vi "JSON Editor.vi"() -> ()   [LabVIEW 2017]
uses:
  Advanced Variant Tools.lvlib
panel:
  in  "reset values to json":bool
  in  "pretty print":bool
  in  "error in (no error)":errorcluster
  in  "update json string":bool
  in  "stop":bool
  in  "JSON String":string
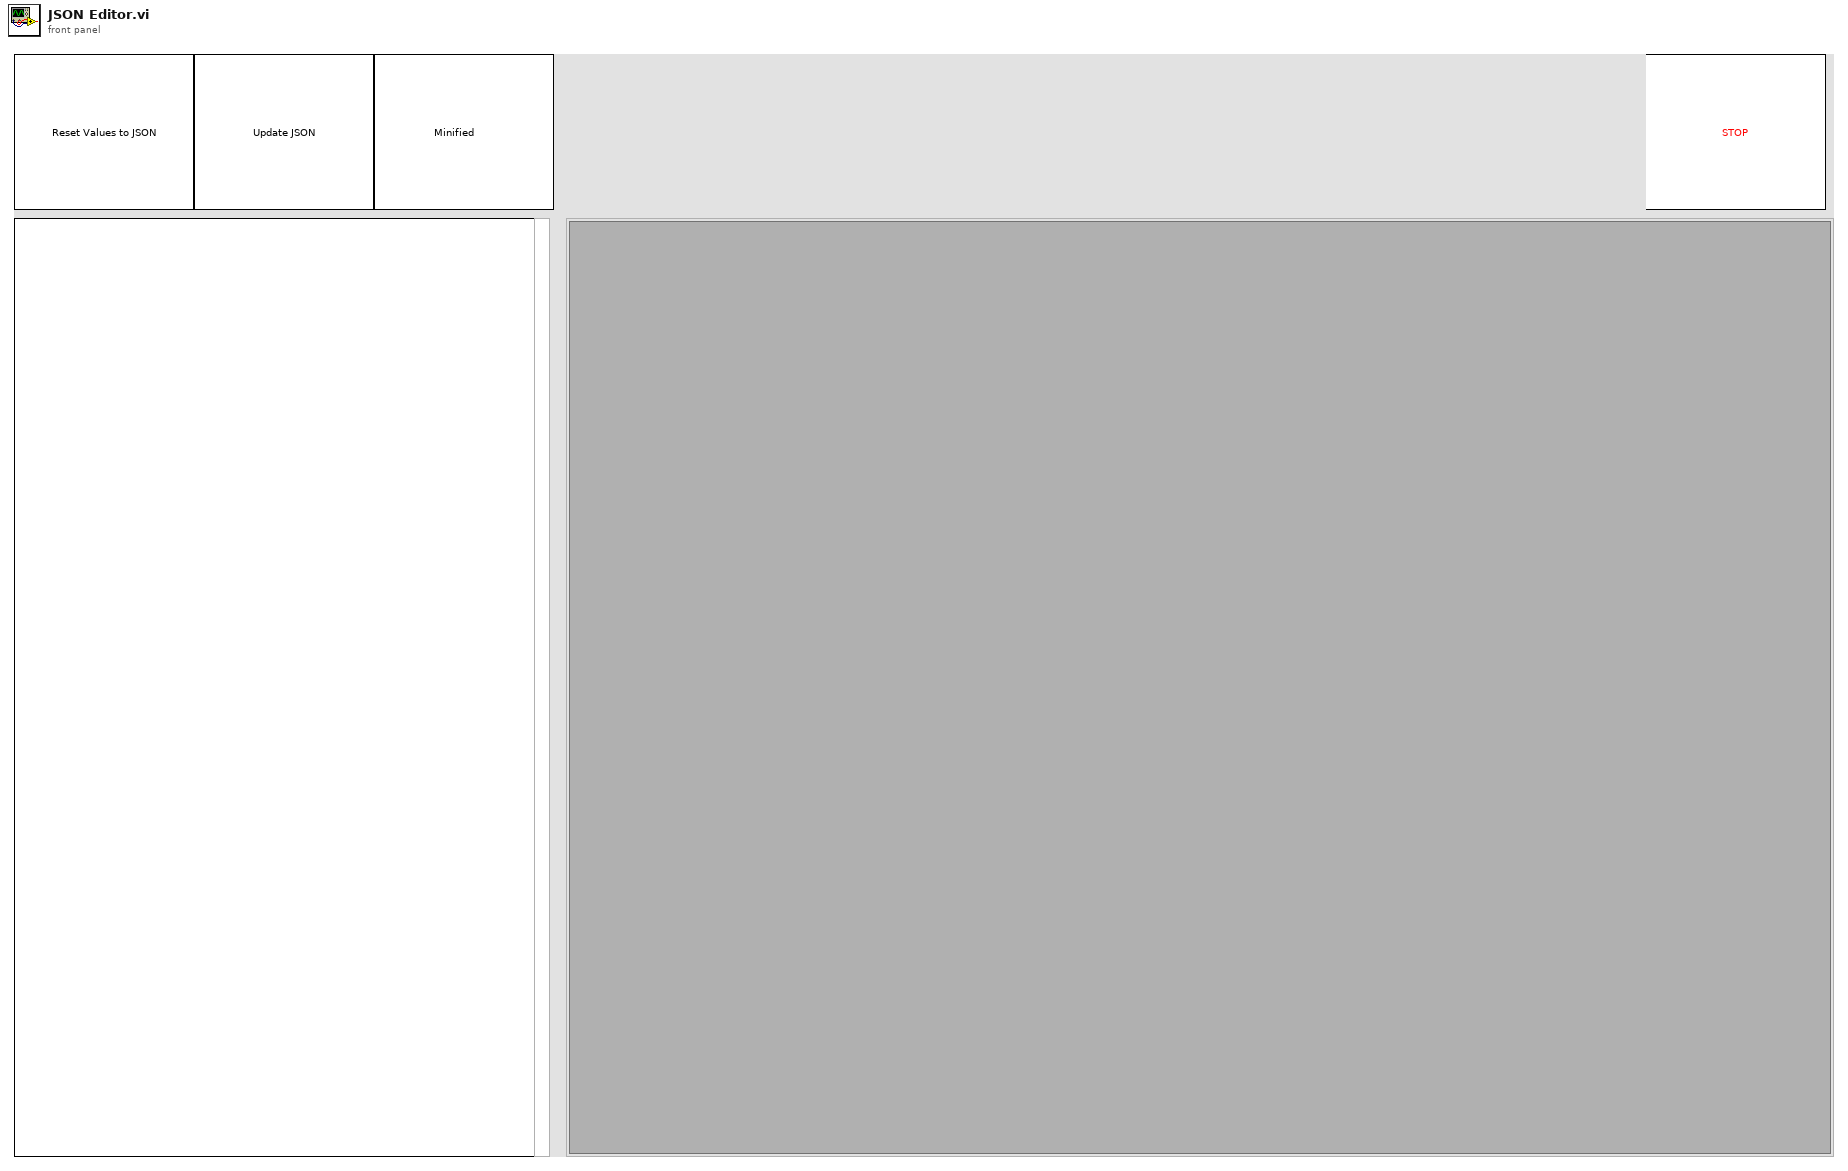
[diagram p1: front panel]
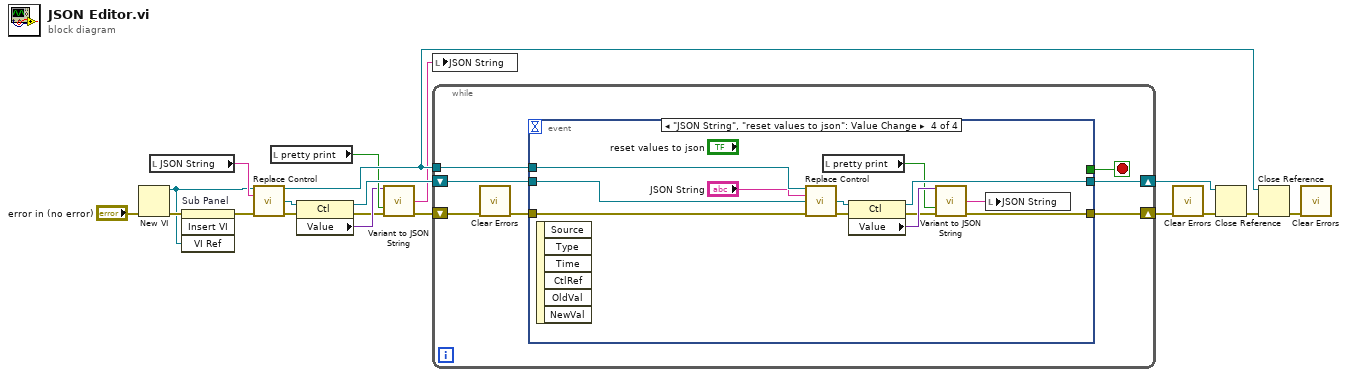
[diagram p0: block diagram]
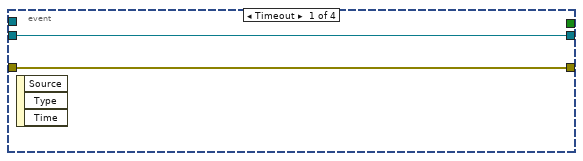
[diagram p2: hidden frame]
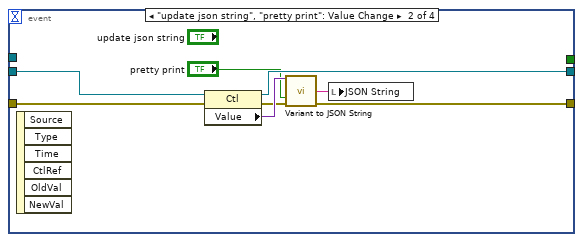
[diagram p3: hidden frame]
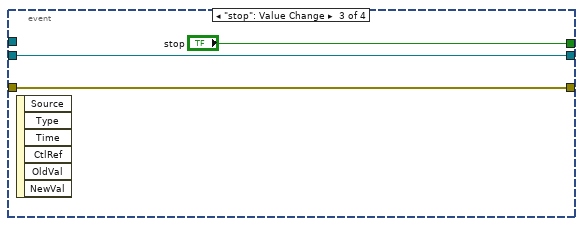
[diagram p4: hidden frame]
diagram:
  n1 = New VI(8:"error in (no error)") -> (0:w15:errorcluster, 3:w14:refnum<vi>)  [unwired: 6 in]
  n2 = local read "JSON String"() -> (w19:string)
  n3 = invoke on="Sub Panel" class="SubPnl" method="Insert VI"(error in=w15, "VI Ref"=w14) -> (error out=w17:errorcluster)  [unwired: 2 in, 3 out]
  n4 = call "Replace Control.vi"("VI in"=w14, "JSON String"=w19, "error in (no error)"=w17) -> ("VI out"=w10:refnum<vi>, "Control out"=w8:refnum<vi>, "error out"=w9:errorcluster)  [unwired: 10 in]
  n5 = local read "pretty print"() -> (w6:bool)
  n6 = property class="Ctl"(reference=w8, error in=w9) -> (reference out=w7:refnum<vi>, error out=w3:errorcluster, "Value"=w5:variant)
  n7 = call "Variant to JSON String.vi"("Variant in"=w5, "pretty print? (F)"=w6, "error in (no error)"=w3) -> ("String"=w4:string, "error out"=w2:errorcluster)  [unwired: 10 in, 1 out]
  n8 = local write "JSON String"(w4) -> ()
  n9 = while {
    shift-right: [w24] -> w13
    shift-left: w2 -> [w25]
    shift-right: [w23] -> w18
    shift-left: w7 -> [w22]
    tunnel: w10 -> [w20]
    stop <- w26 stop-if-true
    n10 = call <vilib>:"Clear Errors.vi"("error in (no error)"=w25) -> ("error out"=w21:errorcluster)  [unwired: 5 in, 1 out]
    n11 = event shown="[3] \"JSON String\", \"reset values to json\": Value Change" {
      selector: _ -> [_ _ _ _]
      dyn-events: _ -> [_ _ _ _]
      timeout: _ -> [_ _ _ _]
      tunnel: [_ _ "stop" _] -> w26
      tunnel: w21 -> [w28 w32 w38 w48]
      tunnel: [w28 w35 w38 w42] -> w24
      tunnel: [w27 w33 w37 w43] -> w23
      tunnel: w22 -> [w27 w34 w37 w50]
      tunnel: w20 -> [_ _ _ w51]
      event Timeout {
        n12 = event-data() -> ()  [unwired: 1 in, 3 out]
      }
      event "update json string", "pretty print": Value Change {
        n13 = event-data() -> ()  [unwired: 1 in, 6 out]
        n14 = property class="Ctl"(reference=w34, error in=w32) -> (reference out=w33:refnum<vi>, error out=w31:errorcluster, "Value"=w36:variant)
        n15 = call "Variant to JSON String.vi"("Variant in"=w36, "pretty print? (F)"="pretty print", "error in (no error)"=w31) -> ("String"=w29:string, "error out"=w35:errorcluster)  [unwired: 10 in, 1 out]
        n16 = local write "JSON String"(w29) -> ()
      }
      event "stop": Value Change {
        n17 = event-data() -> ()  [unwired: 1 in, 6 out]
      }
      event "JSON String", "reset values to json": Value Change {
        n18 = event-data() -> ()  [unwired: 1 in, 6 out]
        n19 = call "Replace Control.vi"("VI in"=w51, "JSON String"="JSON String", "Control in"=w50, "error in (no error)"=w48) -> ("Control out"=w44:refnum<vi>, "error out"=w45:errorcluster)  [unwired: 9 in, 1 out]
        n20 = local read "pretty print"() -> (w41:bool)
        n21 = property class="Ctl"(reference=w44, error in=w45) -> (reference out=w43:refnum<vi>, error out=w46:errorcluster, "Value"=w47:variant)
        n22 = call "Variant to JSON String.vi"("Variant in"=w47, "pretty print? (F)"=w41, "error in (no error)"=w46) -> ("String"=w40:string, "error out"=w42:errorcluster)  [unwired: 10 in, 1 out]
        n23 = local write "JSON String"(w40) -> ()
      }
    }
  }
  n24 = call <vilib>:"Clear Errors.vi"("error in (no error)"=w13) -> ("error out"=w11:errorcluster)  [unwired: 5 in, 1 out]
  n25 = Close Reference(reference=w18, error in (no error)=w11) -> (error out=w12:errorcluster)
  n26 = Close Reference(reference=w10, error in (no error)=w12) -> (error out=w1:errorcluster)
  n27 = call <vilib>:"Clear Errors.vi"("error in (no error)"=w1) -> ()  [unwired: 5 in, 2 out]
